vi "Parse and Format DefinedPulseMap String for Downlink.vi"(9 "Input String":string) -> (2 "Output String":string)   [LabVIEW 2010]
doc: "This VI parses the DefinedPulseMap value from the iput string and formats the data for downlink."
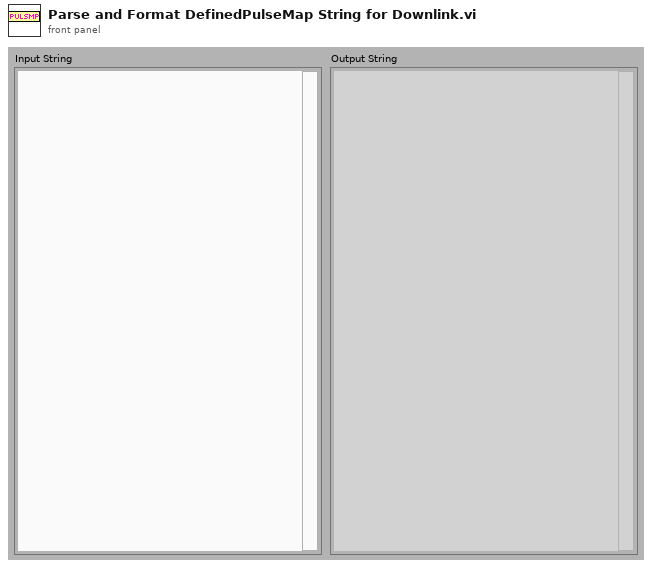
[diagram p1: front panel]
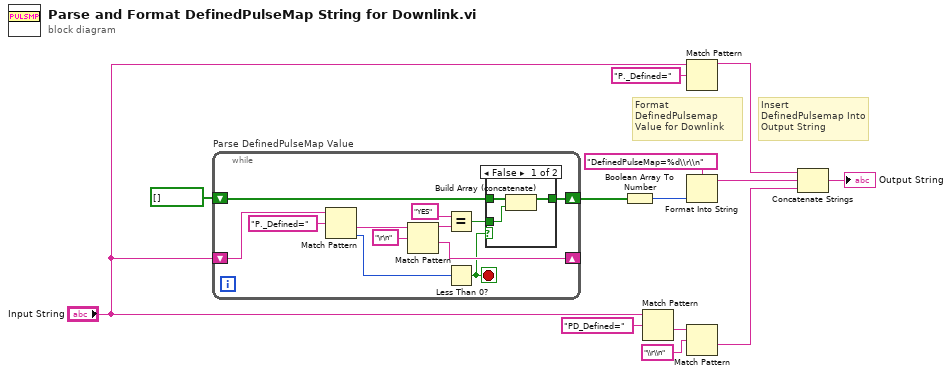
[diagram p0: block diagram]
diagram:
  # "Insert DefinedPulsemap Into Output String"
  # "Format DefinedPulsemap Value for Downlink"
  n1 = while "Parse DefinedPulseMap Value" {
    shift-right: [w22] -> _
    shift-left: "Input String" -> [w25]
    shift-right: [w15] -> w2
    shift-left: bool[] [] -> [w14]
    stop <- w17 stop-if-true
    n2 = Match Pattern(string=w25, regular expression="P._Defined=" ("search string/char (-)")) -> (after substring=w21:string, offset past match=w18:i32)  [unwired: 1 in, 2 out]
    n3 = Match Pattern(string=w21, regular expression="\r\n" ("search string/char (-)")) -> (before substring=w19:string, after substring=w22:string)  [unwired: 1 in, 2 out]
    n4 = Equal?(x="YES", y=w19) -> (x = y?=w16:bool)
    n5 = Less Than 0?(x=w18) -> (x < 0?=w17:bool)
    n6 = case shown="False" w17 {
      tunnel: w16 -> [w28 _]
      tunnel: [w27 w29] -> w15
      tunnel: w14 -> [w26 w29]
      frame False {
        n7 = Build Array (concatenate)(w26, w28) -> (w27:bool[])
      }
      frame True {
      }
    }
  }
  n8 = Boolean Array To Number(Boolean array=w2) -> (number=w11:u32)
  n9 = Match Pattern(string="Input String", regular expression="PD_Defined=" ("search string/char (-)")) -> (after substring=w5:string)  [unwired: 1 in, 3 out]
  n10 = Match Pattern(string="Input String", regular expression="P._Defined=" ("search string/char (-)")) -> (before substring=w8:string)  [unwired: 1 in, 3 out]
  n11 = Format Into String(format string="DefinedPulseMap=%d\\r\\n" ("search string/char (-)"), w11) -> (resulting string=w12:string)  [unwired: 2 in, 1 out]
  n12 = Match Pattern(string=w5, regular expression="\\r\\n") -> (after substring=w9:string)  [unwired: 1 in, 3 out]
  n13 = Concatenate Strings(w8, w12, w9) -> (→"Output String":string)
